vi "Main Tclk.vi"() -> ()   [LabVIEW 2018] (continued)
                    n7612 = local read "FIB time lapse"() -> (w1916:bool)
                    n7613 = case shown="False" w1916 {
                      tunnel: ["FIB imaging paused" ("Status message") "FIB imaging finished" ("Status message")] -> w1917
                      frame True {
                      }
                      frame False {
                      }
                    }
                    n7614 = local write "Status message"(w1917) -> ()
                  }
                }
              }
            }
            n7615 = Add(x=w1864, y=w1865) -> (x+y=w1868:u32)
            n7616 = expression code="x*1000"("FIB time lapse (s)") -> (w1871:u32)
            n7617 = Less?(x=w1868, y=w1871) -> (x < y?=w1867:bool)
            n7618 = Select(t=w1868, s=w1867, f=u32 0) -> (s? t:f=w1870:u32)
          }
        }
        n7619 = Add(x=w1570, y=w1605) -> (x+y=w1610:u32)
        n7620 = local read "Interval (s)"() -> (w1568:u16)
        n7621 = case shown="False" w1546 {
          tunnel: [w1626 w1628] -> w1547
          tunnel: [w1625 w1629] -> w1548
          tunnel: u32 6618880 ("color(black)") -> [w1626 w1629]
          tunnel: u32 16777216 ("color(black)") -> [w1625 w1628]
          tunnel: [w1624 w1627] -> w1540
          frame True {
            n7622 = local read "Median cycle time (s)"() -> (w1624:u32)
          }
          frame False {
            n7623 = local read "Est. cycle time (s)"() -> (w1627:u32)
          }
        }
        n7624 = local read "Milling para"() -> (w1543:T35)
        n7625 = Add(x=w1570, y=w1578) -> (x+y=w1579:u32)
        n7626 = Add(x=w1570, y=w1567) -> (x+y=w1571:u32)
        n7627 = Less?(x=w1610, y=u32 6000) -> (x < y?=w1607:bool)
        n7628 = expression code="x*1000"(w1568) -> (w1569:u16)
        n7629 = Unbundle By Name(w1543) -> ("Z-step (nm)"=w1535:dbl, "Lines auto pause"=w1533:u16)
        n7630 = Less?(x=w1579, y=u32 10000) -> (x < y?=w1582:bool)
        n7631 = Less?(x=w1571, y=w1569) -> (x < y?=w1573:bool)
        n7632 = property on="Median cycle time (s)" class="DigNum (strict)"("Caption.BGColor"=w1547) -> ()  [unwired: 2 in, 2 out]
        n7633 = property on="Est. cycle time (s)" class="DigNum (strict)"("Caption.BGColor"=w1548) -> ()  [unwired: 2 in, 2 out]
        n7634 = expression code="86400/x"(w1540) -> (w1542:u32)
        n7635 = expression code="x/1000"(w1535) -> (w1534:dbl)
        n7636 = Select(t=w1610, s=w1607, f=u32 0) -> (s? t:f=w1606:u32)
        n7637 = Compound Arithmetic op=MULTIPLY(w1542, w1534, w1533) -> (→"Daily Z removal (um)":dbl)
        n7638 = Select(t=w1579, s=w1582, f=u32 0) -> (s? t:f=w1583:u32)
        n7639 = Select(t=w1571, s=w1573, f=u32 0) -> (s? t:f=w1574:u32)
        n7640 = local read "Stop"() -> (w1613:bool)
      }
      n7641 = while {
        stop <- w1175 stop-if-true
        n7642 = Wait Until Next ms Multiple(millisecond multiple=u32 100) -> ()  [unwired: 1 out]
        n7643 = local read "SEM Options"() -> (w1173:T27)
        n7644 = Unbundle By Name(w1173) -> ("Inverse PNG"=w1172:bool)
        n7645 = stacked-sequence {
          tunnel: w1172 -> [_ _ w1232 _]
          frame #0 {
            n7646 = while {
              stop <- w1193 stop-if-true
              n7647 = local read "3D FIB-SEM Files"() -> (w1189:path)
              n7648 = local read "SEM Scan Parameters"() -> (w1183:T26)
              n7649 = Unbundle By Name(w1183) -> ("Y tiles"=w1184:u8, "X tiles"=w1185:u8)
              n7650 = Wait Until Next ms Multiple(millisecond multiple=u32 100) -> ()  [unwired: 1 out]
              n7651 = Decrement(x=w1184) -> (x-1=w1178:u8)
              n7652 = Decrement(x=w1185) -> (x-1=w1177:u8)
              n7653 = Format Into String(w1178) -> (resulting string=w1182:string)  [unwired: 3 in, 1 out]
              n7654 = Format Into String(w1177) -> (resulting string=w1179:string)  [unwired: 3 in, 1 out]
              n7655 = Concatenate Strings("post_" ("name or relative path"), w1182, "-" ("name or relative path"), w1179, ".png" ("name or relative path")) -> (w1181:string)
              n7656 = Build Path(base path=w1189, name or relative path=w1181) -> (appended path=w1190:path)
              n7657 = File/Directory Info(path=w1190) -> (error out=w1191:errorcluster)  [unwired: 1 in, 6 out]
              n7658 = Unbundle By Name(w1191) -> ("status"=w1188:bool)
              n7659 = local read "Stop"() -> (w1192:bool)
              n7660 = Not(x=w1188) -> (.not. x?=w1187:bool)
              n7661 = Or(x=w1187, y=w1192) -> (x .or. y?=w1193:bool)
            }
          }
          frame #1 {
            n7662 = local read "3D FIB-SEM Files"() -> (w1197:path)
            n7663 = local read "SEM Scan Parameters"() -> (w1205:T26)
            n7664 = Unbundle By Name(w1205) -> ("Y tiles"=w1196:u8, "X tiles"=w1195:u8)
            n7665 = Decrement(x=w1196) -> (x-1=w1201:u8)
            n7666 = Decrement(x=w1195) -> (x-1=w1200:u8)
            n7667 = Format Into String(w1201) -> (resulting string=w1204:string)  [unwired: 3 in, 1 out]
            n7668 = Format Into String(w1200) -> (resulting string=w1202:string)  [unwired: 3 in, 1 out]
            n7669 = Concatenate Strings("pre_" ("name or relative path"), w1204, "-" ("name or relative path"), w1202, ".png" ("name or relative path")) -> (w1199:string)
            n7670 = Build Path(base path=w1197, name or relative path=w1199) -> (appended path=w1209:path)
            n7671 = File/Directory Info(path=w1209) -> (error out=w1208:errorcluster)  [unwired: 1 in, 6 out]
            n7672 = Unbundle By Name(w1208) -> ("status"=w1198:bool)
            n7673 = case shown="True" w1198 {
              tunnel: w1197 -> [_ w1212]
              tunnel: w1196 -> [_ w1211]
              tunnel: w1195 -> [_ w1210]
              frame False {
              }
              frame True {
                n7674 = for {
                  N: w1211 -> [_]
                  tunnel: w1212 -> [w1214]
                  tunnel: w1210 -> [w1213]
                  i -> [w1215]
                  n7675 = for {
                    N: w1213 -> [_]
                    tunnel: w1215 -> [w1225]
                    tunnel: w1214 -> [w1216]
                    i -> [w1226]
                    n7676 = Format Into String(w1225) -> (resulting string=w1228:string)  [unwired: 3 in, 1 out]
                    n7677 = Format Into String(w1226) -> (resulting string=w1230:string)  [unwired: 3 in, 1 out]
                    n7678 = Concatenate Strings(w1228, "-" ("name or relative path"), w1230, ".png" ("name or relative path")) -> (w1217:string)
                    n7679 = Concatenate Strings("post_" ("name or relative path"), w1217) -> (w1221:string)
                    n7680 = Concatenate Strings("pre_" ("name or relative path"), w1217) -> (w1222:string)
                    n7681 = Build Path(base path=w1216, name or relative path=w1221) -> (appended path=w1218:path)
                    n7682 = Build Path(base path=w1216, name or relative path=w1222) -> (appended path=w1219:path)
                    n7683 = Move(source path=w1218, 9:TRUE ("overwrite (F)"), 10:w1219) -> ()  [unwired: 2 in, 3 out]
                  }
                }
              }
            }
          }
          frame #2 {
            n7684 = local read "3D FIB-SEM Files"() -> (w1235:path)
            n7685 = local read "SEM Scan Parameters"() -> (w1243:T26)
            n7686 = Unbundle By Name(w1243) -> ("Y tiles"=w1234:u8, "X tiles"=w1233:u8, "Pixel size (nm)"=w1231:sgl)
            n7687 = Decrement(x=w1234) -> (x-1=w1239:u8)
            n7688 = Decrement(x=w1233) -> (x-1=w1238:u8)
            n7689 = Format Into String(w1239) -> (resulting string=w1242:string)  [unwired: 3 in, 1 out]
            n7690 = Format Into String(w1238) -> (resulting string=w1240:string)  [unwired: 3 in, 1 out]
            n7691 = Concatenate Strings("post_" ("name or relative path"), w1242, "-" ("name or relative path"), w1240, ".png" ("name or relative path")) -> (w1237:string)
            n7692 = Build Path(base path=w1235, name or relative path=w1237) -> (appended path=w1247:path)
            n7693 = File/Directory Info(path=w1247) -> (error out=w1246:errorcluster)  [unwired: 1 in, 6 out]
            n7694 = Unbundle By Name(w1246) -> ("status"=w1236:bool)
            n7695 = case shown="False" w1236 {
              tunnel: w1235 -> [w1265 _]
              tunnel: w1234 -> [w1250 _]
              tunnel: w1233 -> [w1249 _]
              tunnel: w1232 -> [w1257 _]
              tunnel: w1231 -> [w1251 _]
              frame False {
                n7696 = for {
                  N: w1250 -> [_]
                  tunnel: w1265 -> [w1272]
                  tunnel: w1249 -> [w1271]
                  tunnel: [w1270] -> w1261 mode=indexing
                  tunnel: [w1269] -> w1260 mode=indexing
                  tunnel: [w1268] -> w1259 mode=indexing
                  tunnel: w1257 -> [w1267]
                  tunnel: [w1266] -> w1256 mode=indexing
                  i -> [w1273]
                  n7697 = for {
                    N: w1271 -> [_]
                    tunnel: w1273 -> [w1290]
                    tunnel: w1272 -> [w1289]
                    tunnel: [w1278] -> w1270 mode=indexing
                    tunnel: [w1275] -> w1269 mode=indexing
                    tunnel: [w1274] -> w1268 mode=indexing
                    tunnel: w1267 -> [w1288]
                    tunnel: [w1287] -> w1266 mode=indexing
                    i -> [w1291]
                    n7698 = Format Into String(w1290) -> (resulting string=w1284:string)  [unwired: 3 in, 1 out]
                    n7699 = Format Into String(w1291) -> (resulting string=w1286:string)  [unwired: 3 in, 1 out]
                    n7700 = Concatenate Strings(w1284, "-" ("name or relative path"), w1286, ".png" ("name or relative path")) -> (w1282:string)
                    n7701 = Concatenate Strings("post_" ("name or relative path"), w1282) -> (w1280:string)
                    n7702 = Concatenate Strings("pre_" ("name or relative path"), w1282) -> (w1279:string)
                    n7703 = call "SIFT align.vi"("post image file"=w1279, "pre image file"=w1280, "Inverse PNG"=w1288, "Affine"=FALSE, "working directory"=w1289) -> ("Delta image"=w1278:dbl, "failed"=w1287:bool, "Delta Y"=w1275:dbl, "Delta X"=w1274:dbl)  [unwired: 1 in, 2 out]
                  }
                }
                "Align failed array" <- w1256
                n7704 = Multiply(x=w1250, y=w1249) -> (x*y=w1248:u8)
                n7705 = Reshape Array(w1259, w1248) -> (w1264:dbl[])
                n7706 = Reshape Array(w1260, w1248) -> (w1263:dbl[])
                n7707 = Reshape Array(w1261, w1248) -> (w1262:dbl[])
                n7708 = call-poly <vilib>:"Mean.vi"("X"=w1264) -> ("mean"=w1255:dbl)  [unwired: 1 out]
                n7709 = call-poly <vilib>:"Mean.vi"("X"=w1263) -> ("mean"=w1253:dbl)  [unwired: 1 out]
                n7710 = call-poly <vilib>:"Mean.vi"("X"=w1262) -> ("mean"=→"Delta image":dbl)  [unwired: 1 out]
                n7711 = Multiply(x=w1255, y=w1251) -> (x*y=→"Delta X":dbl)
                n7712 = Multiply(x=w1253, y=w1251) -> (x*y=→"Delta Y":dbl)
              }
              frame True {
              }
            }
          }
          frame #3 {
            n7713 = local read "3D FIB-SEM Files"() -> (w1294:path)
            n7714 = local read "SEM Scan Parameters"() -> (w1302:T26)
            n7715 = Unbundle By Name(w1302) -> ("Y tiles"=w1293:u8, "X tiles"=w1292:u8)
            n7716 = Decrement(x=w1293) -> (x-1=w1298:u8)
            n7717 = Decrement(x=w1292) -> (x-1=w1297:u8)
            n7718 = Format Into String(w1298) -> (resulting string=w1301:string)  [unwired: 3 in, 1 out]
            n7719 = Format Into String(w1297) -> (resulting string=w1299:string)  [unwired: 3 in, 1 out]
            n7720 = Concatenate Strings("post_" ("name or relative path"), w1301, "-" ("name or relative path"), w1299, ".png" ("name or relative path")) -> (w1296:string)
            n7721 = Build Path(base path=w1294, name or relative path=w1296) -> (appended path=w1306:path)
            n7722 = File/Directory Info(path=w1306) -> (error out=w1305:errorcluster)  [unwired: 1 in, 6 out]
            n7723 = Unbundle By Name(w1305) -> ("status"=w1295:bool)
            n7724 = case shown="False" w1295 {
              tunnel: w1294 -> [w1309 _]
              tunnel: w1293 -> [w1308 _]
              tunnel: w1292 -> [w1307 _]
              frame False {
                n7725 = for {
                  N: w1308 -> [_]
                  tunnel: w1309 -> [w1311]
                  tunnel: w1307 -> [w1310]
                  i -> [w1312]
                  n7726 = for {
                    N: w1310 -> [_]
                    tunnel: w1312 -> [w1322]
                    tunnel: w1311 -> [w1314]
                    i -> [w1323]
                    n7727 = Format Into String(w1322) -> (resulting string=w1325:string)  [unwired: 3 in, 1 out]
                    n7728 = Format Into String(w1323) -> (resulting string=w1327:string)  [unwired: 3 in, 1 out]
                    n7729 = Concatenate Strings(w1325, "-" ("name or relative path"), w1327, ".png" ("name or relative path")) -> (w1313:string)
                    n7730 = Concatenate Strings("post_" ("name or relative path"), w1313) -> (w1318:string)
                    n7731 = Concatenate Strings("pre_" ("name or relative path"), w1313) -> (w1319:string)
                    n7732 = Build Path(base path=w1314, name or relative path=w1318) -> (appended path=w1315:path)
                    n7733 = Build Path(base path=w1314, name or relative path=w1319) -> (appended path=w1316:path)
                    n7734 = Move(source path=w1315, 9:TRUE ("overwrite (F)"), 10:w1316) -> ()  [unwired: 2 in, 3 out]
                  }
                }
              }
              frame True {
              }
            }
          }
        }
        n7735 = local read "Stop"() -> (w1175:bool)
      }
    }
    frame #4 {
      w10117 = sgl[] [] ("FI array")
      w10118 = T44."Enabled" ("Disabled")
      w10129 = FALSE ("Off")
      n7736 = local read "Hardware Configuration"() -> (w10126:T25)
      n7737 = property on="Mill start from Last" class="Bool (strict)"("DisabledEnum"=w10118) -> ()  [unwired: 2 in, 2 out]
      n7738 = local write "Stop"(w10129) -> ()
      n7739 = local write "Off"(w10129) -> ()
      n7740 = local write "3D FIB-SEM"(w10129) -> ()
      n7741 = local write "Scan x1"(w10129) -> ()
      n7742 = local write "Scan xn"(w10129) -> ()
      n7743 = local write "FIB time lapse"(w10129) -> ()
      n7744 = property on="Scan x1" class="Bool (strict)"("DisabledEnum"=w10118) -> ()  [unwired: 2 in, 2 out]
      n7745 = property on="Scan xn" class="Bool (strict)"("DisabledEnum"=w10118) -> ()  [unwired: 2 in, 2 out]
      n7746 = property on="FIB Imaging" class="Bool (strict)"("DisabledEnum"=w10118) -> ()  [unwired: 2 in, 2 out]
      n7747 = property on="FIB time lapse" class="Bool (strict)"("DisabledEnum"=w10118) -> ()  [unwired: 2 in, 2 out]
      n7748 = property on="Reset" class="Bool (strict)"("DisabledEnum"=w10118) -> ()  [unwired: 2 in, 2 out]
      n7749 = property on="Pre image" class="Bool (strict)"("DisabledEnum"=w10118) -> ()  [unwired: 2 in, 2 out]
      n7750 = property on="Post image" class="Bool (strict)"("DisabledEnum"=w10118) -> ()  [unwired: 2 in, 2 out]
      n7751 = shared-variable "My Computer\\Zeiss Library.lvlib\\Stop"(w10129) -> ()  [unwired: 1 in, 1 out]
      n7752 = Unbundle By Name(w10126) -> ("SEM X coil"=w10121:refnum<k15>, "SEM Y coil"=w10120:refnum<k15>, "SEM Detectors"=w10119:refnum<k15>)
      n7753 = property on="FIB Profile" class="Bool (strict)"("DisabledEnum"=w10118) -> ()  [unwired: 2 in, 2 out]
      n7754 = property on="Start Current DataLog" class="Bool (strict)"("DisabledEnum"=w10118) -> ()  [unwired: 2 in, 2 out]
      n7755 = property on="Beam blanked" class="Bool (strict)"("DisabledEnum"=w10118) -> ()  [unwired: 2 in, 2 out]
      n7756 = property on="Spot" class="Bool (strict)"("DisabledEnum"=w10118) -> ()  [unwired: 2 in, 2 out]
      n7757 = property on="ROI" class="Bool (strict)"("DisabledEnum"=w10118) -> ()  [unwired: 2 in, 2 out]
      n7758 = property on="Mill Stop" class="Bool (strict)"("DisabledEnum"=w10118) -> ()  [unwired: 2 in, 2 out]
      n7759 = property on="Mill" class="Bool (strict)"("DisabledEnum"=w10118) -> ()  [unwired: 2 in, 2 out]
      n7760 = property on="FIB FOV (um)" class="DigNum (strict)"("DisabledEnum"=w10118) -> ()  [unwired: 2 in, 2 out]
      n7761 = property on="X resolution" class="DigNum (strict)"("DisabledEnum"=w10118) -> ()  [unwired: 2 in, 2 out]
      n7762 = property on="Z resolution" class="DigNum (strict)"("DisabledEnum"=w10118) -> ()  [unwired: 2 in, 2 out]
      n7763 = property on="Z-step (nm)" class="DigNum (strict)"("DisabledEnum"=w10118) -> ()  [unwired: 2 in, 2 out]
      n7764 = property on="X center (um)" class="DigNum (strict)"("DisabledEnum"=w10118) -> ()  [unwired: 2 in, 2 out]
      n7765 = property on="Z center (um)" class="DigNum (strict)"("DisabledEnum"=w10118) -> ()  [unwired: 2 in, 2 out]
      n7766 = property on="X size (um)" class="DigNum (strict)"("DisabledEnum"=w10118) -> ()  [unwired: 2 in, 2 out]
      n7767 = property on="Z size (um)" class="DigNum (strict)"("DisabledEnum"=w10118) -> ()  [unwired: 2 in, 2 out]
      n7768 = Build Array(w10121, w10120) -> (w10122:refnum<k15>[])
      n7769 = call <instrlib>:"niScope Abort.vi"("instrument handle"=w10119) -> ("instrument handle out"=w10124:refnum<k15>, "error out"=w10123:errorcluster)  [unwired: 13 in]
      n7770 = call <instrlib>:"niScope Close.vi"("instrument handle"=w10124, "error in"=w10123) -> ("error out"=w10125:errorcluster)  [unwired: 13 in]
      n7771 = local read "Machine Type"() -> (w10127:u8)
      n7772 = for {
        tunnel: w10122 -> [w10134] mode=indexing
        shift-right: [w10131] -> _
        shift-left: w10125 -> [w10133]
        n7773 = call <instrlib>:"niFgen Abort Generation.vi"("error in (no error)"=w10133, "Instrument Handle"=w10134) -> ("error out"=w10132:errorcluster, "Instrument Handle Out"=w10130:refnum<k15>)  [unwired: 8 in]
        n7774 = call <instrlib>:"niFgen Close.vi"("error in (no error)"=w10132, "Instrument Handle"=w10130) -> ("error out"=w10131:errorcluster)  [unwired: 9 in]
      }
      n7775 = local write "Faraday Cup array"(w10117) -> ()
      n7776 = local write "SEM Specimen I array"(w10117) -> ()
      n7777 = local write "Beam Dump 1 array"(w10117) -> ()
      n7778 = local write "Beam Dump 2 array"(w10117) -> ()
      n7779 = local write "Milling I array"(w10117) -> ()
      n7780 = local write "Focus index array"(w10117) -> ()
      n7781 = local write "FRC array"(w10117) -> ()
      n7782 = local write "Delta Z array"(w10117) -> ()
      n7783 = local write "Delta X sum array"(w10117) -> ()
      n7784 = local write "Delta Y sum array"(w10117) -> ()
      n7785 = local write "Delta image array"(w10117) -> ()
      n7786 = local write "Milling Z voltage array"(w10117) -> ()
      n7787 = local write "Re-engage Delta X array"(w10117) -> ()
      n7788 = local write "Re-engage Delta Y array"(w10117) -> ()
      n7789 = local write "Re-engage X shift array"(w10117) -> ()
      n7790 = local write "Re-engage Y shift array"(w10117) -> ()
      n7791 = local write "Specimen I array"(w10117) -> ()
      n7792 = local write "FI grid array tiled"(sgl[][][][][] [] ("FI grid array tiled")) -> ()
      n7793 = local write "FI array"(w10117) -> ()
      n7794 = local write "Temp array"(w10117) -> ()
      n7795 = local write "Delta X array"(w10117) -> ()
      n7796 = local write "Delta Y array"(w10117) -> ()
      n7797 = case shown="2" w10127 {
        frame 0, Default {
        }
        frame 2 {
          n7798 = local read "Api"() -> (w10141:refnum<k7>)
          n7799 = call "SmartSEM Remote API set float.vi"("vValue"=sgl 0.0, "lpszParam"="DP_PANEL_DISABLE", "ActiveX Container"=w10141) -> ("error out"=w10135:errorcluster, "reference out"=w10137:refnum<k7>)  [unwired: 7 in]
          n7800 = call "SmartSEM Remote API set float.vi"("error in"=w10135, "vValue"=sgl 0.0, "lpszParam"="DP_JOYSTICK_DISABLE", "ActiveX Container"=w10137) -> ()  [unwired: 6 in, 2 out]
        }
      }
      n7801 = local write "Temp high limit array"(w10117) -> ()
      n7802 = local write "Temp low limit array"(w10117) -> ()
      n7803 = local write "Specimen I high limit array"(w10117) -> ()
      n7804 = local write "Specimen I low limit array"(w10117) -> ()
      n7805 = local write "SEM Specimen I high limit array"(w10117) -> ()
      n7806 = local write "SEM Specimen I low limit array"(w10117) -> ()
      n7807 = local write "FI low limit array"(w10117) -> ()
      n7808 = local write "Faraday Cup high limit array"(w10117) -> ()
      n7809 = local write "Faraday Cup low limit array"(w10117) -> ()
      n7810 = local write "BD1 high limit array"(w10117) -> ()
      n7811 = local write "BD1 low limit array"(w10117) -> ()
      n7812 = local write "BD2 high limit array"(w10117) -> ()
      n7813 = local write "BD2 low limit array"(w10117) -> ()
      n7814 = local write "Milling I high limit array"(w10117) -> ()
      n7815 = local write "Milling I low limit array"(w10117) -> ()
    }
  }
